vi "Windowed Data.vi"(8 "CrsrList":T1, 9 "Waveform in":waveform(dbl)) -> (1 "Windowed\nPeriod (Td)":dbl, 2 "Spectral\nResolution (Fd)":dbl, 3 "Windowed num. of samples 2":dbl)   [LabVIEW 2014, in "Aquisicao de Dados.lvlib"]
uses:
  Aquisicao de Dados.lvlib
  <vilib>/Utility/miscctls.llb/LVCursorListTypeDef.ctl
  <vilib>/Waveform/WDTOps.llb/WDT Number of Waveform Samples DBL.vi
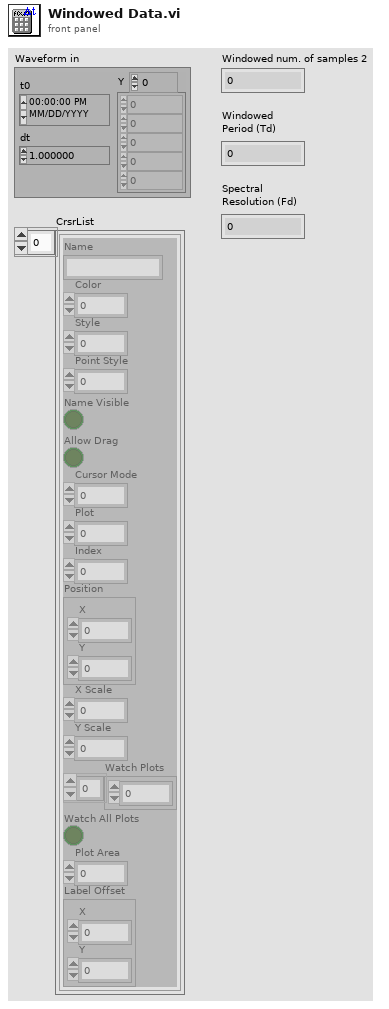
[diagram p1: front panel]
types:
  T1 = typedef "LVCursorListTypeDef.ctl" = cluster{"Name":string, "Color":u32, "Style":u8, "Point Style":u8, "Name Visible":bool, "Allow Drag":bool, "Cursor Mode":u32, "Plot":i32, "Index":i32, "Position":cluster{"X":dbl, "Y":dbl}, "X Scale":u32, "Y Scale":u32, "Watch Plots":i32[], "Watch All Plots":bool, "Plot Area":i32, "Label Offset":cluster{"X":dbl, "Y":dbl}}[]
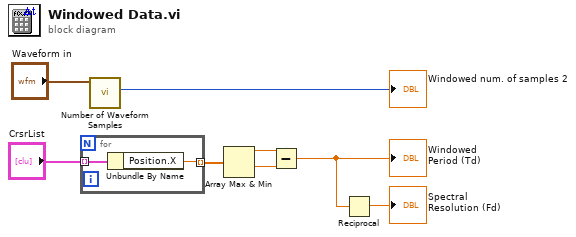
[diagram p0: block diagram]
diagram:
  n1 = for {
    tunnel: "CrsrList" -> [w10] mode=indexing
    tunnel: [w9] -> w3 mode=indexing
    n2 = Unbundle By Name(w10) -> ("Position.X"=w9:dbl)
  }
  n3 = call-poly <vilib>:"Number of Waveform Samples.vi"("waveform in"="Waveform in") -> ("number of samples"=→"Windowed num. of samples 2":i32)  [unwired: 8 in, 2 out]
  n4 = Array Max & Min(array=w3) -> (max value=w5:dbl, min value=w6:dbl)  [unwired: 2 out]
  n5 = Subtract(x=w5, y=w6) -> (x-y=w8:dbl)
  "Windowed\nPeriod (Td)" <- w8
  n6 = Reciprocal(x=w8) -> (1/x=→"Spectral\nResolution (Fd)":dbl)
